vi "assets.property.set.vi"   [LabVIEW 2020]
uses:
  asset.lvclass
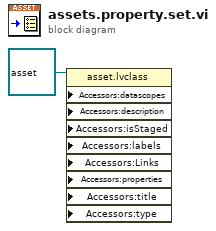
[diagram p0: block diagram]
diagram:
  n1 = property class="asset.lvclass" props=["Accessors:datascopes", "Accessors:description", "Accessors:isStaged", "Accessors:labels", "Accessors:Links", "Accessors:properties", "Accessors:title", "Accessors:type"](reference=refnum<class "asset.lvclass"> refnum ("asset.lvclass")) -> ()  [unwired: 9 in, 2 out]
